vi "Bind Insert Command Values.vi"(8 "Error In (no error)":errorcluster, 10 "Record":variant, 11 "SQL Statement In":refnum<class "SQL Statement.lvclass">) -> (0 "Error Out":errorcluster, 3 "SQL Statement Out":refnum<class "SQL Statement.lvclass">)   [LabVIEW 2023, in "SQLite DB Operator.lvclass"]
uses:
  SQLite DB Operator.lvclass
  SQLite DB Operator.lvclass/SQLite DB Operator.ctl
  DB Records/Expenses Tracker Record/Public/Ctrls/Category.ctl
  DB Records/Expenses Tracker Record/Expenses Tracker Record.lvclass
  <vilib>/drjdpowell/SQLite Library/SQL Statement/SQL Statement.lvclass
  <vilib>/Utility/Data Type/NI_Data Type.lvlib
  DB Records/Expenses Tracker Record/Public/Ctrls/Transaction.ctl
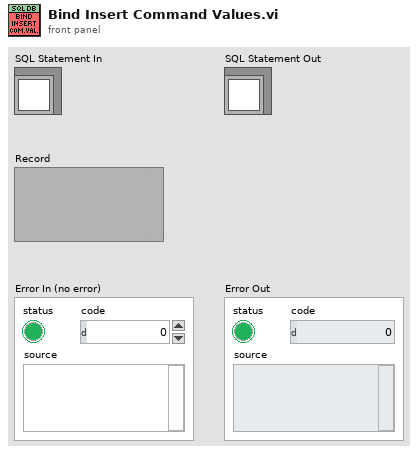
[diagram p1: front panel]
types:
  T1 = typedef "Expenses Tracker Record.lvclass/Category.ctl" = cluster{"ID":u32, "Name":string}
  T2 = typedef "Expenses Tracker Record.lvclass/Transaction.ctl" = cluster{"ID":u32, "Name":string, "Is Income":bool, "Value":dbl, "Amount":dbl, "Total":dbl, "Date of Entry":timestamp, "Date":timestamp, "Last Update":timestamp, "Category":u32, "Subcategory":u32, "Cycle":u32, "Description":string}
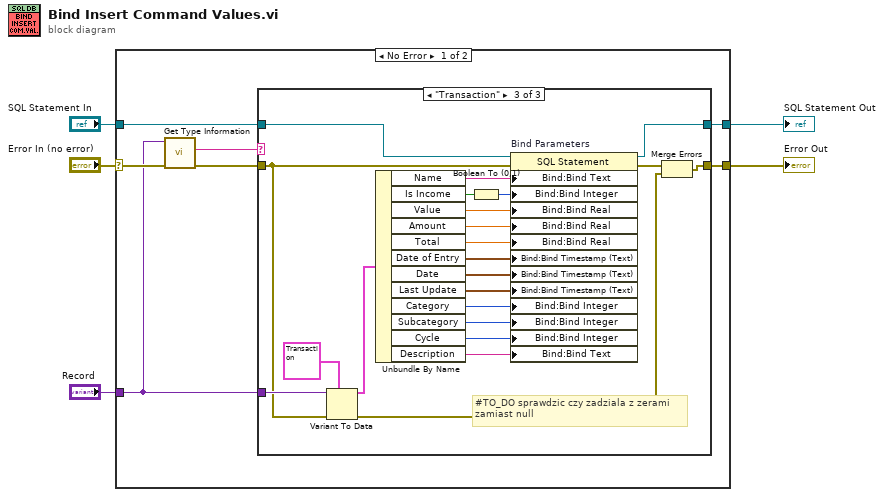
[diagram p0: block diagram]
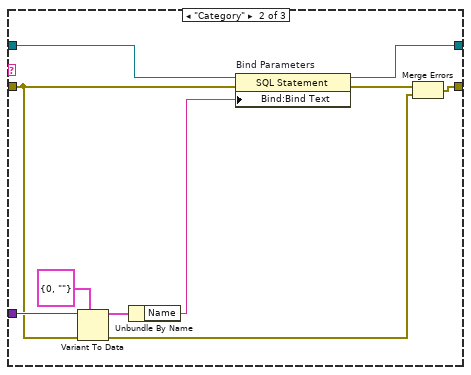
[diagram p3: hidden frame]
diagram:
  n1 = case shown="No Error" "Error In (no error)" {
    selector: "Error In (no error)" -> [w9 w47]
    tunnel: "SQL Statement In" -> [w12 w48]
    tunnel: [w11 w47] -> w4
    tunnel: [w10 w48] -> w3
    tunnel: "Record" -> [w8 _]
    frame No Error {
      n2 = call <vilib>:"Get Type Information.vi"("error in (no error)"=w9, "variant"=w8) -> ("error out"=w6:errorcluster, "name"=w7:string)  [unwired: 5 in, 3 out]
      n3 = case shown="\"Transaction\"" w7 {
        tunnel: w8 -> [_ w24 w46]
        tunnel: [w13 w23 w45] -> w10
        tunnel: [w14 w16 w38] -> w11
        tunnel: w12 -> [w13 w21 w43]
        tunnel: w6 -> [w14 w17 w39]
        frame Default {
        }
        frame "Category" {
          n4 = Variant To Data(error in=w17, type=T1 {"ID"=0, "Name"=""} ("Category"), Variant=w24) -> (data=w20:T1, error out=w15:errorcluster)
          n5 = Unbundle By Name(w20) -> ("Name"=w18:string)
          n6 = property on="Bind Parameters" class="SQL Statement"(reference=w21, error in=w17, "Bind:Bind Text"=w18) -> (reference out=w23:refnum<class "SQL Statement.lvclass">, error out=w22:errorcluster)
          n7 = Merge Errors(w22, w15) -> (w16:errorcluster)
        }
        frame "Transaction" {
          # "#TO_DO sprawdzic czy zadziala z zerami\nzamiast null"
          n8 = Variant To Data(error in=w39, type=T2 {"ID"=0, "Name"="", "Is Income"=FALSE, "Value"=0.0, "Amount"=0.0, "Total"=0.0, "Date of Entry"=timestamp(0 s since 1904-01-01), "Date"=timestamp(0 s since 1904-01-01), "Last Update"=timestamp(0 s since 1904-01-01), "Category"=0, "Subcategory"=0, "Cycle"=0, "Description"=""} ("Transaction"), Variant=w46) -> (data=w42:T2, error out=w37:errorcluster)
          n9 = Unbundle By Name(w42) -> ("Name"=w40:string, "Is Income"=w26:bool, "Value"=w34:dbl, "Amount"=w35:dbl, "Total"=w36:dbl, "Date of Entry"=w33:timestamp, "Date"=w32:timestamp, "Last Update"=w31:timestamp, "Category"=w27:u32, "Subcategory"=w28:u32, "Cycle"=w29:u32, "Description"=w30:string)
          n10 = Boolean To (0,1)(Boolean=w26) -> (0, 1=w25:i16)
          n11 = property on="Bind Parameters" class="SQL Statement"(reference=w43, error in=w39, "Bind:Bind Text"=w40, "Bind:Bind Integer"=w25, "Bind:Bind Real"=w34, "Bind:Bind Real"=w35, "Bind:Bind Real"=w36, "Bind:Bind Timestamp (Text)"=w33, "Bind:Bind Timestamp (Text)"=w32, "Bind:Bind Timestamp (Text)"=w31, "Bind:Bind Integer"=w27, "Bind:Bind Integer"=w28, "Bind:Bind Integer"=w29, "Bind:Bind Text"=w30) -> (reference out=w45:refnum<class "SQL Statement.lvclass">, error out=w44:errorcluster)
          n12 = Merge Errors(w44, w37) -> (w38:errorcluster)
        }
      }
    }
    frame Error {
    }
  }
  "Error Out" <- w4
  "SQL Statement Out" <- w3
